vi "Updater Read Installed Spartan Version.vi"(6 "DEBUG? (f)":bool, 7 "Version Control Name\n(\"Version\")":string="Version", 8 "error in (no error)":errorcluster, 9 "Version Global\n(\"Spartan Version.vi\")":string="Spartan Version.vi", 10 "Library Name (Spartan Common.llb)":string="Spartan Common.llb", 11 "Spartan Install Folder (empty)":path) -> (0 "error out":errorcluster, 2 "Version":T1 {"Build Date/Time" format="%<%X\n%x>T"}, 3 "dup Spartan Install Folder":path)   [LabVIEW 2011]
uses:
  SI.LIB/OGAB Version.ctl
  SI.LIB/WIN32/WinSHELL/SHFolderPaths.ctl
  OpenG.LIB/file/file.llb/Valid Path - Traditional__ogtk.vi
panel:
  # "Leave this control empty to find\nthe \"Program Files\\Summitek\\Spartan\"\ndirectory from the Windows API..."
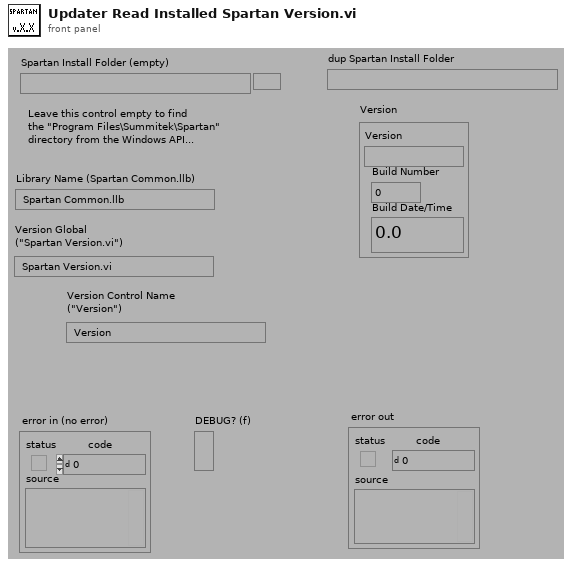
[diagram p1: front panel]
types:
  T1 = typedef "OGAB Version.ctl" = cluster{"Version":string, "Build Number":u32, "Build Date/Time":dbl}
  T2 = typedef "SHFolderPaths.ctl" = i32
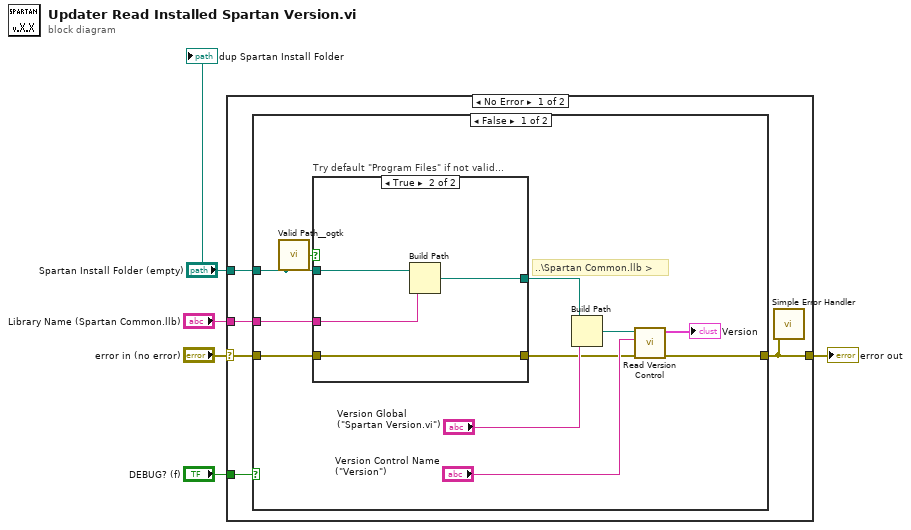
[diagram p0: block diagram]
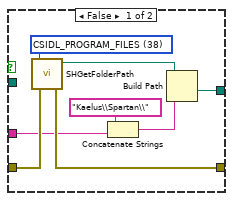
[diagram p2: hidden frame]
diagram:
  n1 = case shown="No Error" "error in (no error)" {
    selector: "error in (no error)" -> [w6 w35]
    tunnel: "Library Name (Spartan Common.llb)" -> [w10 _]
    tunnel: "Spartan Install Folder (empty)" -> [w9 _]
    tunnel: "DEBUG? (f)" -> [w8 _]
    tunnel: [w7 w35] -> w2
    frame No Error {
      n2 = case shown="False" w8 {
        tunnel: w6 -> [w21 w34]
        tunnel: w10 -> [w20 _]
        tunnel: [w11 w34] -> w7
        tunnel: w9 -> [w14 _]
        frame False {
          # "..\\Spartan Common.llb >"
          n3 = call-poly "Valid Path__ogtk.vi"("path"=w14) -> ("valid"=w15:bool)
          n4 = case "Try default \"Program Files\" if not valid..." shown="True" w15 {
            tunnel: w21 -> [w28 w33]
            tunnel: [w27 w33] -> w13
            tunnel: w20 -> [w25 w31]
            tunnel: w14 -> [_ w32]
            tunnel: [w22 w30] -> w18
            frame False {
              w29 = T2 38 items=["CSIDL_DESKTOP"=0, "CSIDL_PERSONAL"=5, "CSIDL_STARTUP"=7, "CSIDL_BITBUCKET"=10, "CSIDL_DRIVES"=17, "CSIDL_NETWORK"=18, "CSIDL_COMMON_PROGRAMS"=23, "CSIDL_COMMON_STARTUP"=24, "CSIDL_COMMON_DESKTOPDIRECTORY"=25, "CSIDL_PROGRAM_FILES"=38] ("Shell Folder (DESKTOP)")
              n5 = call "SHGetFolderPath.vi"("error in (no error)"=w28, "Shell Folder (DESKTOP)"=w29) -> ("error out"=w27:errorcluster, "FolderPath"=w26:path)  [unwired: 4 out]
              n6 = Concatenate Strings("Kaelus\\Spartan\\", w25) -> (w23:string)
              n7 = Build Path(base path=w26, name or relative path=w23) -> (appended path=w22:path)
            }
            frame True {
              n8 = Build Path(base path=w32, name or relative path=w31) -> (appended path=w30:path)
            }
          }
          n9 = Build Path(base path=w18, name or relative path="Version Global\n(\"Spartan Version.vi\")") -> (appended path=w19:path)
          n10 = call "Read Version Control.vi"("error in (no error)"=w13, "Version Control Name (\"Version\")"="Version Control Name\n(\"Version\")", "Path to Version Global (empty)"=w19) -> ("error out"=w11:errorcluster, "Version"=→"Version":T1)  [unwired: 3 out]
        }
        frame True {
        }
      }
      n11 = call <vilib>:"Simple Error Handler.vi"("error in (no error)"=w7) -> ()  [unwired: 4 in, 5 out]
    }
    frame Error {
    }
  }
  "error out" <- w2
  "dup Spartan Install Folder" <- "Spartan Install Folder (empty)"
